vi "AUTOMAT.vi"() -> ()   [LabVIEW 2014]
uses:
  Timer 2013/Control Timer.ctl
  <vilib>/Platform/TimedLoop/XDataNode/timing_clust.ctl
  <vilib>/Platform/TimedLoop/XDataNode/nitl_modes.ctl
  <vilib>/Platform/TimedLoop/XDataNode/wakeup.ctl
  <vilib>/platform/TimedLoop/XDataNode/XDataNode.xnode
  <vilib>/Platform/TimedLoop/XDataNode/XDNodeRunTimeDep.lvlib
panel:
  out "Siren":bool
  out "B4":bool
  out "B1":bool
  out "B2":bool
  out "B3":bool
  out "B5":bool
  out "Ventil":bool
  out "SISTEM":bool
  out "PUMPE":bool
  out "Pump 2":bool
  out "Pump 1":bool
  in  "GENERAL STOP":bool
  in  "RUCNO/AUTOMATSKI":bool
  in  "Accept Stop":bool
  out "SYSTEM STOPPED":bool
  in  "Pumpe OFF":bool
  in  "Pumpe ON":bool
  in  "Sistem OFF":bool
  in  "Sistem ON":bool
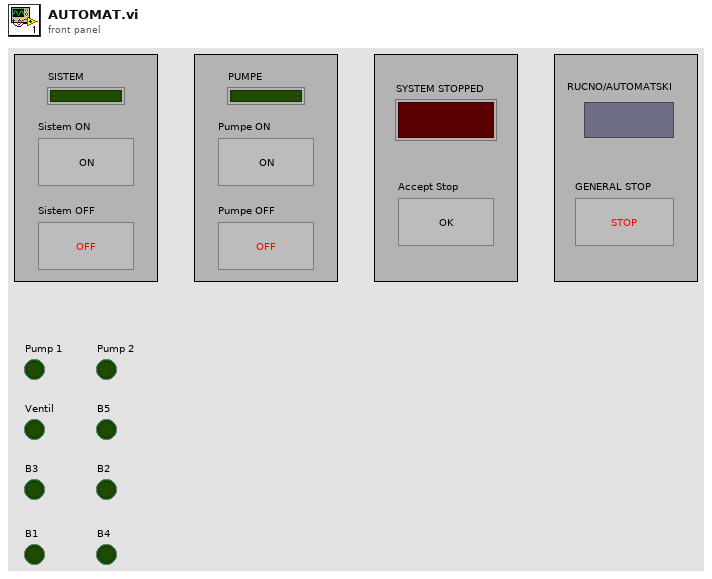
[diagram p1: front panel]
types:
  T1 = typedef "Control Timer.ctl" = enum16{"Timecheck", "Reset"}
  T2 = typedef "XDNodeRunTimeDep.lvlib/timing_clust.ctl" = cluster{"Expected End [f-1]":u64, "Actual End [f-1]":u64, "Finished Late? [f-1]":bool, "Expected End [i-1]":u64, "Actual End [i-1]":u64, "Finished Late? [i-1]":bool, "Expected Start [i]":u64, "Actual Start [i]":u64, "Expected Start [f]":u64, "Actual Start [f]":u64, "Source Name":string, "Structure Name":string, "Period":i64, "Deadline":i64, "Offset":i64, "Start":i64, "Priority":i32, "Timeout":i32, "Mode":T3, "Wakeup Reason":T4, "Error":errorcluster, "Source Type":string, "Secondary Source Type":string, "Global End Time":u64, "Global Start Time":u64, "Frame Duration":u64, "Iteration Duration":u64, "Assigned CPU":i32, "I/O Scan Engine Mode":u32}
  T3 = typedef "XDNodeRunTimeDep.lvlib/nitl_modes.ctl" = enum32{"No Change", "Process missed periods, maintain original phase", "Discard missed periods, maintain original phase", "Process missed periods, ignore original phase", "Discard missed periods, ignore original phase"}
  T4 = typedef "XDNodeRunTimeDep.lvlib/wakeup.ctl" = enum32{"Normal", "Aborted", "Asynchronous wakeup", "Timing source error", "Timed loop error", "Timeout"}
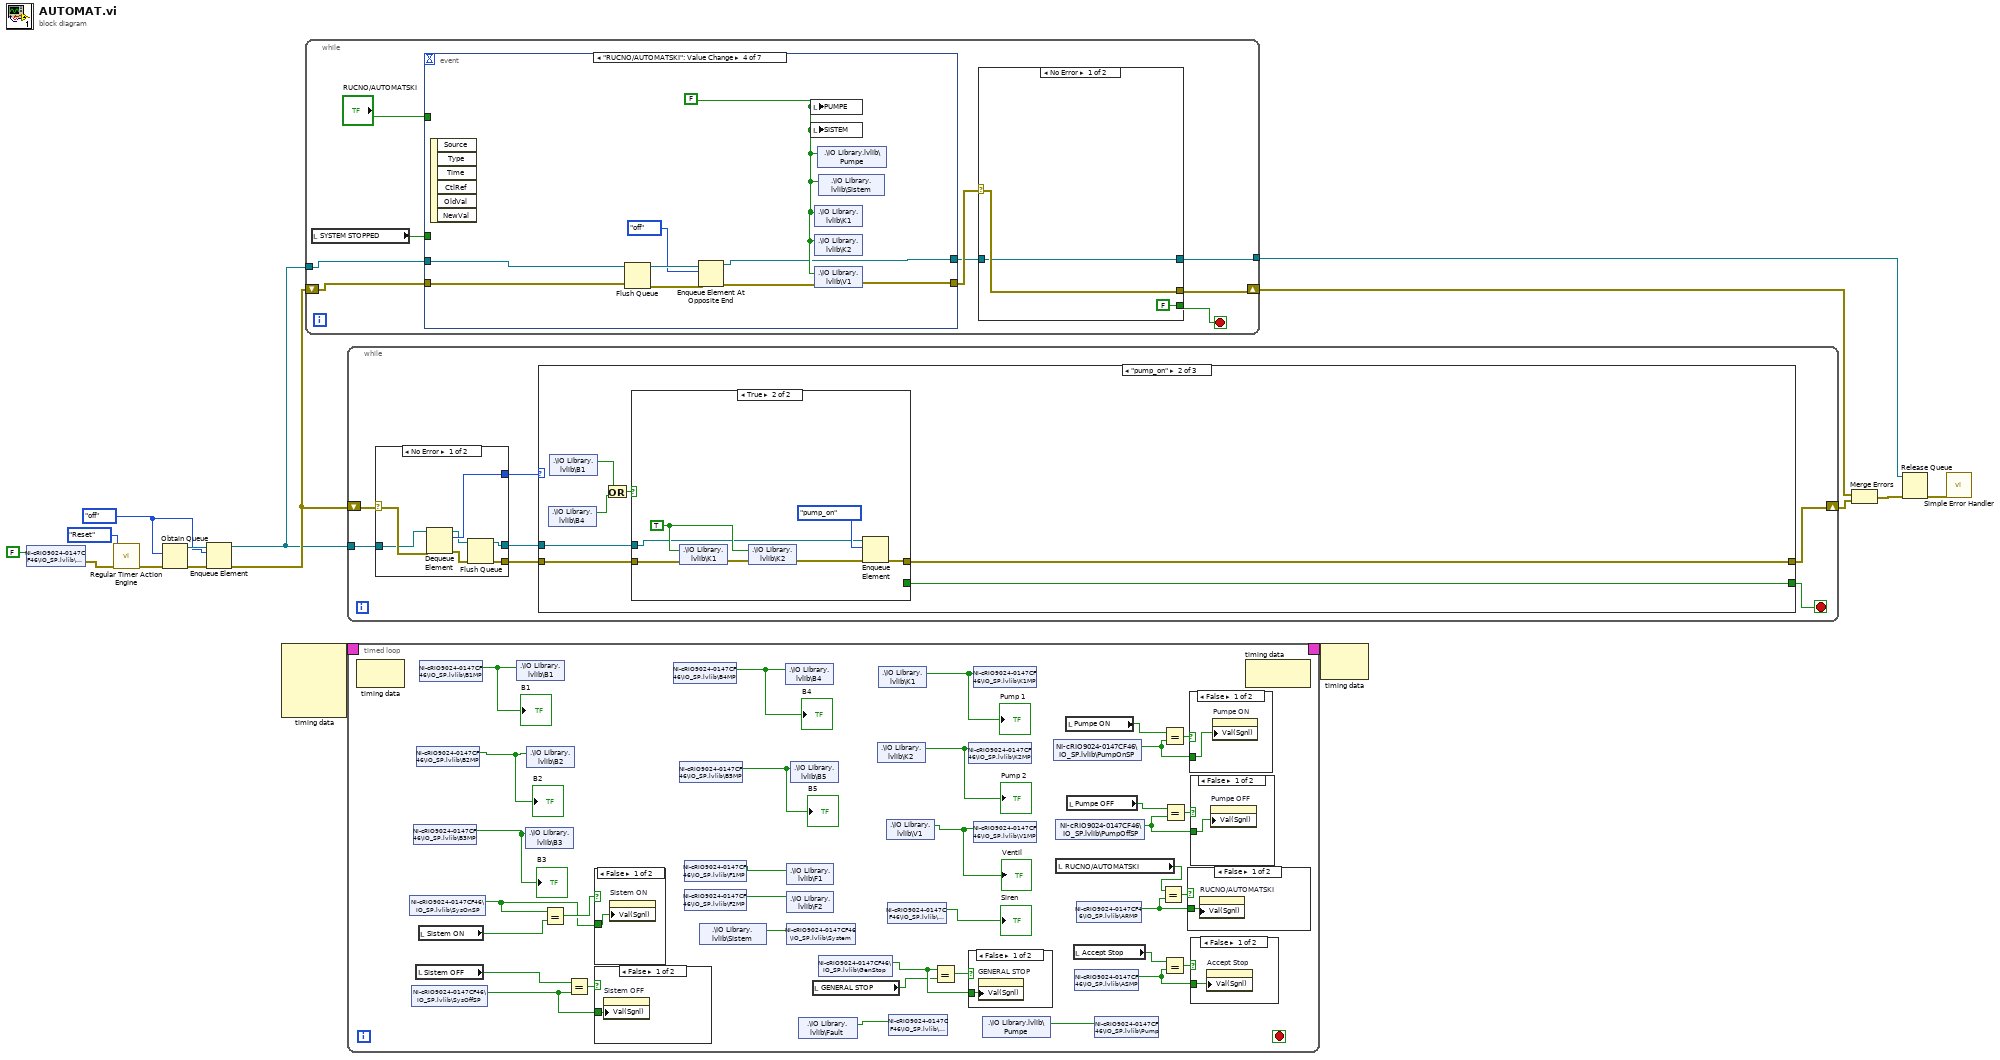
[diagram p0: block diagram]
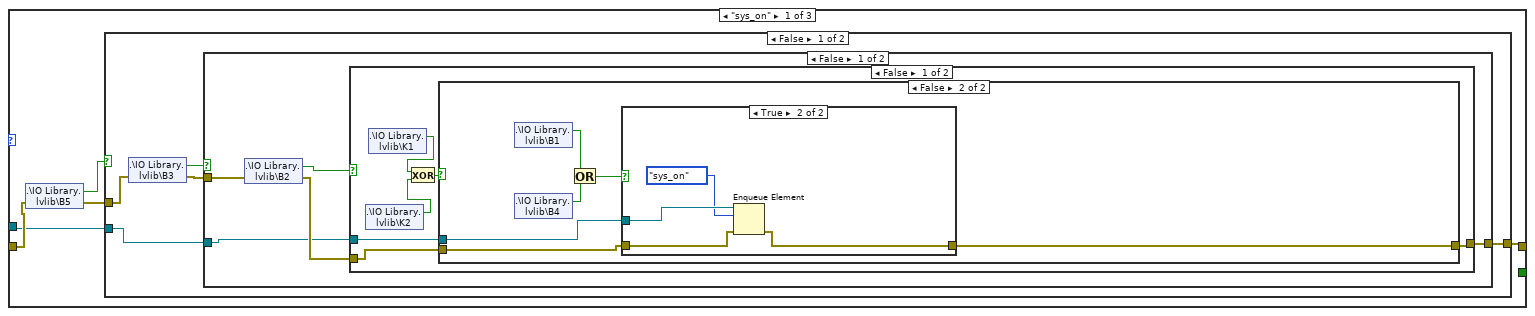
[diagram p9: hidden frame]
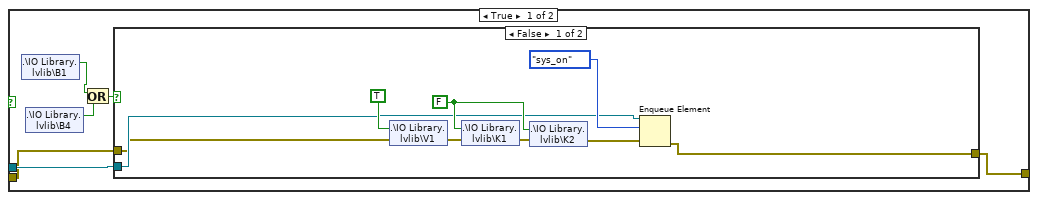
[diagram p10: hidden frame]
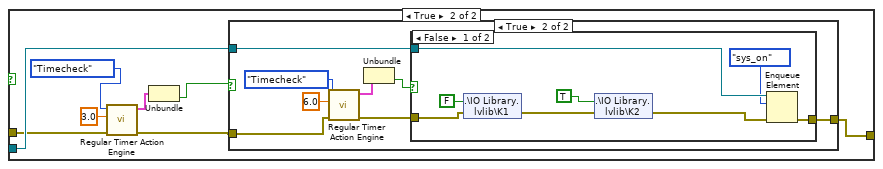
[diagram p11: hidden frame]
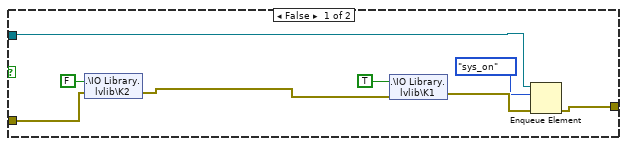
[diagram p12: hidden frame]
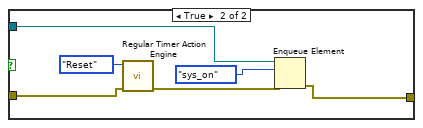
[diagram p13: hidden frame]
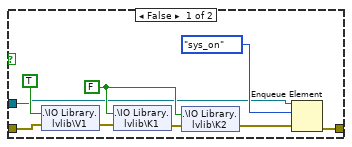
[diagram p14: hidden frame]
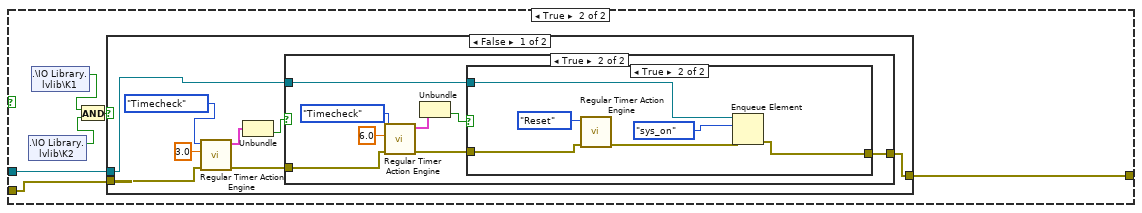
[diagram p15: hidden frame]
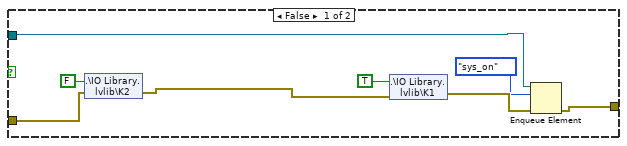
[diagram p16: hidden frame]
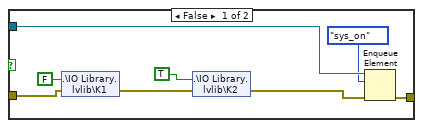
[diagram p17: hidden frame]
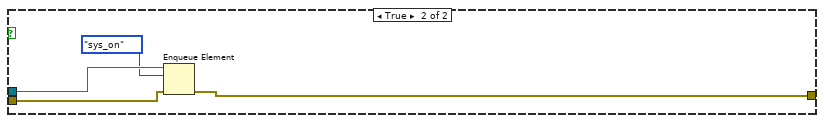
[diagram p18: hidden frame]
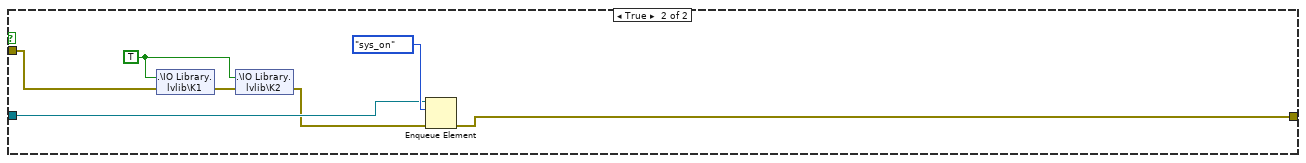
[diagram p19: hidden frame]
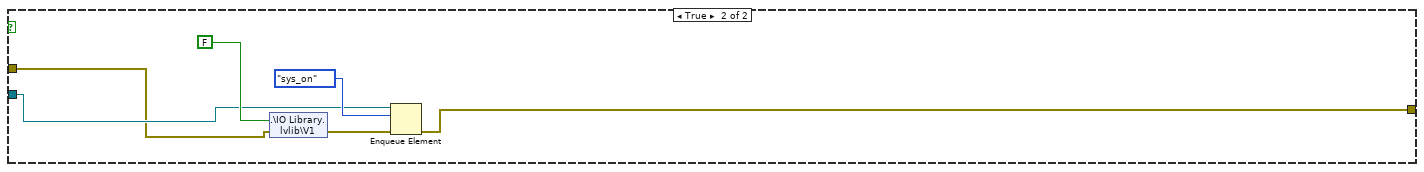
[diagram p20: hidden frame]
diagram:
  w14 = enum16{"sys_on", "pump_on", "off"}."off" ("Enum")
  n1 = shared-variable "NI-cRIO9024-0147CF46\\IO_SP.lvlib\\Siren"(FALSE ("Siren")) -> (error out=w2:errorcluster)  [unwired: 1 in]
  n2 = call "Regular Timer Action Engine.vi"("Enum"=Control_Timer."Reset", "error in"=w2) -> ("error out"=w11:errorcluster)  [unwired: 7 in, 1 out]
  n3 = Obtain Queue(element data type=w14, error in (no error)=w11) -> (queue out=w15:refnum<queue>, error out=w16:errorcluster)  [unwired: 3 in, 1 out]
  n4 = Enqueue Element(queue=w15, element=w14, error in (no error)=w16) -> (queue out=w12:refnum<queue>, error out=w13:errorcluster)  [unwired: 1 in, 1 out]
  n5 = node-c288() -> (w4:T2)  [unwired: 4 in]
  n6 = while {
    tunnel: w12 -> [w17]
    shift-right: [w25] -> w8
    shift-left: w13 -> [w18]
    tunnel: [w20] -> w9
    stop <- w24 stop-if-true
    n7 = local read "SYSTEM STOPPED"() -> (w21:bool)
    n8 = event shown="[3] \"RUCNO/AUTOMATSKI\": Value Change" {
      selector: _ -> [_ _ _ _ _ _ _]
      dyn-events: _ -> [_ _ _ _ _ _ _]
      timeout: _ -> [_ _ _ _ _ _ _]
      tunnel: "RUCNO/AUTOMATSKI" -> [w31 _ _ _ w85 w109 w126]
      tunnel: w18 -> [w30 w51 w61 w79 w83 w107 w124]
      tunnel: w17 -> [w29 w49 w70 w78 w82 w106 w125]
      tunnel: [w28 w52 w64 w77 w84 w108 w123] -> w22
      tunnel: w21 -> [w27 _ _ _ w81 _ _]
      tunnel: [w26 w50 w66 w73 w80 w105 w122] -> w19
      event "Pumpe ON": Value Change {
        n9 = event-data() -> ()  [unwired: 1 in, 6 out]
        n10 = case shown="False" w27 {
          tunnel: w31 -> [_ w38]
          tunnel: w30 -> [w33 w37]
          tunnel: w29 -> [w32 w36]
          tunnel: [w33 w35] -> w28
          tunnel: [w32 w34] -> w26
          frame True {
          }
          frame False {
            n11 = case shown="False" w38 {
              tunnel: w37 -> [w39 w48]
              tunnel: w36 -> [w40 w47]
              tunnel: [w39 w44] -> w35
              tunnel: [w40 w45] -> w34
              frame True {
              }
              frame False {
                w46 = TRUE ("Pump 2 contactor")
                n12 = Flush Queue(queue=w47, error in (no error)=w48) -> (queue out=w42:refnum<queue>, error out=w41:errorcluster)  [unwired: 1 out]
                n13 = shared-variable ".\\IO Library.lvlib\\K1"(w46) -> ()  [unwired: 1 in, 1 out]
                n14 = shared-variable ".\\IO Library.lvlib\\K2"(w46) -> ()  [unwired: 1 in, 1 out]
                n15 = shared-variable ".\\IO Library.lvlib\\Pumpe"(w46) -> ()  [unwired: 1 in, 1 out]
                n16 = Enqueue Element At Opposite End(queue=w42, element=enum16{"sys_on", "pump_on", "off"}."pump_on", error in (no error)=w41) -> (queue out=w45:refnum<queue>, error out=w44:errorcluster)  [unwired: 1 in, 1 out]
                "PUMPE" <- w46
              }
            }
          }
        }
      }
      event "Accept Stop": Value Change {
        n17 = event-data() -> ()  [unwired: 1 in, 6 out]
        n18 = local read "GENERAL STOP"() -> (w53:bool)
        n19 = case shown="False" w53 {
          tunnel: [w54 w59] -> w52
          tunnel: w51 -> [w55 w59]
          tunnel: [w57 w58] -> w50
          tunnel: w49 -> [w57 w58]
          frame False {
            w56 = FALSE ("SYSTEM STOPPED")
            n20 = shared-variable ".\\IO Library.lvlib\\Fault"(w56, error in=w55) -> (error out=w54:errorcluster)
            "SYSTEM STOPPED" <- w56
          }
          frame True {
          }
        }
      }
      event "GENERAL STOP": Value Change {
        w60 = FALSE
        w63 = TRUE ("SYSTEM STOPPED")
        n21 = event-data() -> ()  [unwired: 1 in, 6 out]
        n22 = shared-variable ".\\IO Library.lvlib\\Fault"(w63, error in=w61) -> (error out=w62:errorcluster)
        n23 = local write "SYSTEM STOPPED"(w63) -> ()
        n24 = Flush Queue(queue=w70, error in (no error)=w62) -> (queue out=w68:refnum<queue>, error out=w69:errorcluster)  [unwired: 1 out]
        n25 = Enqueue Element At Opposite End(queue=w68, element=enum16{"sys_on", "pump_on", "off"}."off", error in (no error)=w69) -> (queue out=w66:refnum<queue>, error out=w65:errorcluster)  [unwired: 1 in, 1 out]
        n26 = shared-variable ".\\IO Library.lvlib\\Pumpe"(w60) -> ()  [unwired: 1 in, 1 out]
        n27 = shared-variable ".\\IO Library.lvlib\\Sistem"(w60) -> ()  [unwired: 1 in, 1 out]
        n28 = local write "SISTEM"(w60) -> ()
        n29 = local write "PUMPE"(w60) -> ()
        n30 = shared-variable ".\\IO Library.lvlib\\K1"(w60) -> ()  [unwired: 1 in, 1 out]
        n31 = shared-variable ".\\IO Library.lvlib\\K2"(w60) -> ()  [unwired: 1 in, 1 out]
        n32 = shared-variable ".\\IO Library.lvlib\\V1"(w60) -> ()  [unwired: 1 in, 1 out]
        n33 = shared-variable "NI-cRIO9024-0147CF46\\IO_SP.lvlib\\Siren"(w60, error in=w65) -> (error out=w64:errorcluster)
      }
      event "RUCNO/AUTOMATSKI": Value Change {
        w76 = FALSE
        n34 = event-data() -> ()  [unwired: 1 in, 6 out]
        n35 = Flush Queue(queue=w78, error in (no error)=w79) -> (queue out=w74:refnum<queue>, error out=w75:errorcluster)  [unwired: 1 out]
        n36 = Enqueue Element At Opposite End(queue=w74, element=enum16{"sys_on", "pump_on", "off"}."off", error in (no error)=w75) -> (queue out=w73:refnum<queue>, error out=w72:errorcluster)  [unwired: 1 in, 1 out]
        n37 = local write "PUMPE"(w76) -> ()
        n38 = local write "SISTEM"(w76) -> ()
        n39 = shared-variable ".\\IO Library.lvlib\\K1"(w76) -> ()  [unwired: 1 in, 1 out]
        n40 = shared-variable ".\\IO Library.lvlib\\K2"(w76) -> ()  [unwired: 1 in, 1 out]
        n41 = shared-variable ".\\IO Library.lvlib\\V1"(w76, error in=w72) -> (error out=w77:errorcluster)
        n42 = shared-variable ".\\IO Library.lvlib\\Pumpe"(w76) -> ()  [unwired: 1 in, 1 out]
        n43 = shared-variable ".\\IO Library.lvlib\\Sistem"(w76) -> ()  [unwired: 1 in, 1 out]
      }
      event "Sistem ON": Value Change {
        n44 = event-data() -> ()  [unwired: 1 in, 6 out]
        n45 = case shown="False" w81 {
          tunnel: w85 -> [_ w92]
          tunnel: [w87 w91] -> w84
          tunnel: w83 -> [w87 w90]
          tunnel: w82 -> [w86 w89]
          tunnel: [w86 w88] -> w80
          frame True {
          }
          frame False {
            n46 = case shown="True" w92 {
              tunnel: [w93 w99] -> w91
              tunnel: w90 -> [w93 w95]
              tunnel: w89 -> [w94 w98]
              tunnel: [w94 w100] -> w88
              frame False {
              }
              frame True {
                w97 = TRUE ("V1")
                n47 = shared-variable ".\\IO Library.lvlib\\Sistem"(w97, error in=w95) -> (error out=w96:errorcluster)
                n48 = shared-variable ".\\IO Library.lvlib\\V1"(w97, error in=w96) -> (error out=w104:errorcluster)
                n49 = Flush Queue(queue=w98, error in (no error)=w104) -> (queue out=w102:refnum<queue>, error out=w103:errorcluster)  [unwired: 1 out]
                n50 = Enqueue Element At Opposite End(queue=w102, element=enum16{"sys_on", "pump_on", "off"}."sys_on", error in (no error)=w103) -> (queue out=w100:refnum<queue>, error out=w99:errorcluster)  [unwired: 1 in, 1 out]
                "SISTEM" <- w97
              }
            }
          }
        }
      }
      event "Sistem OFF": Value Change {
        n51 = event-data() -> ()  [unwired: 1 in, 6 out]
        n52 = case shown="True" w109 {
          tunnel: [w110 w116] -> w108
          tunnel: w107 -> [w110 w112]
          tunnel: w106 -> [w111 w115]
          tunnel: [w111 w117] -> w105
          frame False {
          }
          frame True {
            w114 = FALSE ("V1")
            n53 = shared-variable ".\\IO Library.lvlib\\Sistem"(w114, error in=w112) -> (error out=w113:errorcluster)
            n54 = local write "SISTEM"(w114) -> ()
            n55 = shared-variable ".\\IO Library.lvlib\\V1"(w114, error in=w113) -> (error out=w121:errorcluster)
            n56 = Flush Queue(queue=w115, error in (no error)=w121) -> (queue out=w119:refnum<queue>, error out=w120:errorcluster)  [unwired: 1 out]
            n57 = Enqueue Element At Opposite End(queue=w119, element=enum16{"sys_on", "pump_on", "off"}."off", error in (no error)=w120) -> (queue out=w117:refnum<queue>, error out=w116:errorcluster)  [unwired: 1 in, 1 out]
          }
        }
      }
      event "Pumpe OFF": Value Change {
        n58 = event-data() -> ()  [unwired: 1 in, 6 out]
        n59 = case shown="False" w126 {
          tunnel: w125 -> [w128 w134]
          tunnel: w124 -> [w127 w135]
          tunnel: [w127 w133] -> w123
          tunnel: [w128 w132] -> w122
          frame True {
          }
          frame False {
            w129 = FALSE ("Pump 1 contactor")
            n60 = Flush Queue(queue=w134, error in (no error)=w135) -> (queue out=w137:refnum<queue>, error out=w138:errorcluster)  [unwired: 1 out]
            n61 = Enqueue Element At Opposite End(queue=w137, element=enum16{"sys_on", "pump_on", "off"}."off", error in (no error)=w138) -> (queue out=w132:refnum<queue>, error out=w136:errorcluster)  [unwired: 1 in, 1 out]
            n62 = local write "PUMPE"(FALSE ("PUMPE")) -> ()
            n63 = shared-variable ".\\IO Library.lvlib\\K1"(w129, error in=w136) -> (error out=w131:errorcluster)
            n64 = shared-variable ".\\IO Library.lvlib\\Pumpe"(w129, error in=w131) -> (error out=w130:errorcluster)
            n65 = shared-variable ".\\IO Library.lvlib\\K2"(w129, error in=w130) -> (error out=w133:errorcluster)
          }
        }
      }
    }
    n66 = case shown="No Error" w22 {
      selector: w22 -> [w143 w146]
      tunnel: [w143 w146] -> w25
      tunnel: [FALSE TRUE] -> w24
      tunnel: [w141 w144] -> w20
      tunnel: w19 -> [w141 w144]
      frame No Error {
      }
      frame Error {
      }
    }
  }
  n67 = while {
    shift-right: [w148] -> w7
    shift-left: w13 -> [w153]
    tunnel: w12 -> [w152]
    stop <- w147 stop-if-true
    n68 = case shown="No Error" w153 {
      selector: w153 -> [w342 w345]
      tunnel: w152 -> [w341 w343]
      tunnel: [w340 enum16{"sys_on", "pump_on", "off"}."off" ("Enum")] -> w151
      tunnel: [w339 w345] -> w150
      tunnel: [w338 w343] -> w149
      frame No Error {
        n69 = Dequeue Element(queue=w341, error in (no error)=w342) -> (queue out=w337:refnum<queue>, element=w340:enum16{"sys_on", "pump_on", "off"}, error out=w336:errorcluster)  [unwired: 1 in, 1 out]
        n70 = Flush Queue(queue=w337, error in (no error)=w336) -> (queue out=w338:refnum<queue>, error out=w339:errorcluster)  [unwired: 1 out]
      }
      frame Error {
      }
    }
    n71 = case shown="\"pump_on\"" w151 {
      tunnel: [w155 w313 w332] -> w148
      tunnel: w150 -> [w157 w312 w328]
      tunnel: w149 -> [w154 w309 w331]
      tunnel: [_ w308 _] -> w147
      frame "sys_on" {
        n72 = shared-variable ".\\IO Library.lvlib\\B5"(error in=w157) -> (w158:bool, error out=w156:errorcluster)
        n73 = case shown="False" w158 {
          tunnel: w156 -> [w163 w303]
          tunnel: [w161 w302] -> w155
          tunnel: w154 -> [w160 w304]
          frame False {
            n74 = shared-variable ".\\IO Library.lvlib\\B3"(error in=w163) -> (w162:bool, error out=w159:errorcluster)
            n75 = case shown="False" w162 {
              tunnel: [w166 w300] -> w161
              tunnel: w160 -> [w164 w299]
              tunnel: w159 -> [w167 w298]
              frame False {
                n76 = shared-variable ".\\IO Library.lvlib\\B2"(error in=w167) -> (w168:bool, error out=w165:errorcluster)
                n77 = case shown="False" w168 {
                  tunnel: [w174 w248] -> w166
                  tunnel: w165 -> [w172 w249]
                  tunnel: w164 -> [w173 w247]
                  frame False {
                    n78 = shared-variable ".\\IO Library.lvlib\\K2"() -> (w169:bool)  [unwired: 1 in, 1 out]
                    n79 = shared-variable ".\\IO Library.lvlib\\K1"() -> (w170:bool)  [unwired: 1 in, 1 out]
                    n80 = Exclusive Or(1:w169, 2:w170) -> (0:w171:bool)
                    n81 = case shown="False" w171 {
                      tunnel: [w180 w230] -> w174
                      tunnel: w173 -> [w176 w229]
                      tunnel: w172 -> [w175 w228]
                      frame True {
                        n82 = shared-variable ".\\IO Library.lvlib\\B1"() -> (w178:bool)  [unwired: 1 in, 1 out]
                        n83 = shared-variable ".\\IO Library.lvlib\\B4"() -> (w177:bool)  [unwired: 1 in, 1 out]
                        n84 = Or(x=w178, y=w177) -> (x .or. y?=w179:bool)
                        n85 = case shown="False" w179 {
                          tunnel: [w181 w192] -> w180
                          tunnel: w176 -> [w186 w191]
                          tunnel: w175 -> [w185 w190]
                          frame False {
                            w187 = FALSE
                            n86 = shared-variable ".\\IO Library.lvlib\\V1"(TRUE, error in=w185) -> (error out=w184:errorcluster)
                            n87 = shared-variable ".\\IO Library.lvlib\\K1"(w187, error in=w184) -> (error out=w183:errorcluster)
                            n88 = shared-variable ".\\IO Library.lvlib\\K2"(w187, error in=w183) -> (error out=w182:errorcluster)
                            n89 = Enqueue Element(queue=w186, element=enum16{"sys_on", "pump_on", "off"}."sys_on", error in (no error)=w182) -> (error out=w181:errorcluster)  [unwired: 1 in, 2 out]
                          }
                          frame True {
                            n90 = call "Regular Timer Action Engine.vi"("Enum"=Control_Timer."Timecheck", "Time Target"=3.0, "error in"=w190) -> ("Status"=w195:cluster{"Running":bool, "Done":bool}, "error out"=w193:errorcluster)  [unwired: 6 in]
                            n91 = Unbundle(w195) -> ("Done"=w194:bool)  [unwired: 1 out]
                            n92 = case shown="True" w194 {
                              tunnel: w193 -> [w204 w211]
                              tunnel: [w203 w207] -> w192
                              tunnel: w191 -> [w201 w206]
                              frame False {
                                n93 = shared-variable ".\\IO Library.lvlib\\K2"(FALSE ("F2"), error in=w204) -> (error out=w199:errorcluster)
                                n94 = shared-variable ".\\IO Library.lvlib\\K1"(TRUE ("Pump 2 contactor"), error in=w199) -> (error out=w202:errorcluster)
                                n95 = Enqueue Element(queue=w201, element=enum16{"sys_on", "pump_on", "off"}."sys_on", error in (no error)=w202) -> (error out=w203:errorcluster)  [unwired: 1 in, 2 out]
                              }
                              frame True {
                                n96 = call "Regular Timer Action Engine.vi"("Enum"=Control_Timer."Timecheck", "Time Target"=6.0, "error in"=w211) -> ("Status"=w210:cluster{"Running":bool, "Done":bool}, "error out"=w208:errorcluster)  [unwired: 6 in]
                                n97 = Unbundle(w210) -> ("Done"=w209:bool)  [unwired: 1 out]
                                n98 = case shown="False" w209 {
                                tunnel: w208 -> [w216 w227]
                                tunnel: [w220 w224] -> w207
                                tunnel: w206 -> [w219 w223]
                                frame False {
                                n99 = shared-variable ".\\IO Library.lvlib\\K1"(FALSE ("K1"), error in=w216) -> (error out=w215:errorcluster)
                                n100 = shared-variable ".\\IO Library.lvlib\\K2"(TRUE ("Pump 2 contactor"), error in=w215) -> (error out=w214:errorcluster)
                                n101 = Enqueue Element(queue=w219, element=enum16{"sys_on", "pump_on", "off"}."sys_on", error in (no error)=w214) -> (error out=w220:errorcluster)  [unwired: 1 in, 2 out]
                                }
                                frame True {
                                n102 = call "Regular Timer Action Engine.vi"("Enum"=Control_Timer."Reset", "error in"=w227) -> ("error out"=w225:errorcluster)  [unwired: 7 in, 1 out]
                                n103 = Enqueue Element(queue=w223, element=enum16{"sys_on", "pump_on", "off"}."sys_on", error in (no error)=w225) -> (error out=w224:errorcluster)  [unwired: 1 in, 2 out]
                                }
                                }
                              }
                            }
                          }
                        }
                      }
                      frame False {
                        n104 = shared-variable ".\\IO Library.lvlib\\B1"() -> (w232:bool)  [unwired: 1 in, 1 out]
                        n105 = shared-variable ".\\IO Library.lvlib\\B4"() -> (w231:bool)  [unwired: 1 in, 1 out]
                        n106 = Or(x=w232, y=w231) -> (x .or. y?=w233:bool)
                        n107 = case shown="True" w233 {
                          tunnel: w228 -> [w240 w246]
                          tunnel: [w242 w245] -> w230
                          tunnel: w229 -> [w234 w244]
                          frame False {
                            w235 = FALSE
                            n108 = shared-variable ".\\IO Library.lvlib\\V1"(TRUE, error in=w240) -> (error out=w238:errorcluster)
                            n109 = shared-variable ".\\IO Library.lvlib\\K1"(w235, error in=w238) -> (error out=w236:errorcluster)
                            n110 = shared-variable ".\\IO Library.lvlib\\K2"(w235, error in=w236) -> (error out=w237:errorcluster)
                            n111 = Enqueue Element(queue=w234, element=enum16{"sys_on", "pump_on", "off"}."sys_on", error in (no error)=w237) -> (error out=w242:errorcluster)  [unwired: 1 in, 2 out]
                          }
                          frame True {
                            n112 = Enqueue Element(queue=w244, element=enum16{"sys_on", "pump_on", "off"}."sys_on", error in (no error)=w246) -> (error out=w245:errorcluster)  [unwired: 1 in, 2 out]
                          }
                        }
                      }
                    }
                  }
                  frame True {
                    n113 = shared-variable ".\\IO Library.lvlib\\K2"() -> (w250:bool)  [unwired: 1 in, 1 out]
                    n114 = shared-variable ".\\IO Library.lvlib\\K1"() -> (w251:bool)  [unwired: 1 in, 1 out]
                    n115 = And(x=w251, y=w250) -> (x .and. y?=w252:bool)
                    n116 = case shown="False" w252 {
                      tunnel: w249 -> [w257 w294]
                      tunnel: [w254 w293] -> w248
                      tunnel: w247 -> [w253 w292]
                      frame False {
                        n117 = call "Regular Timer Action Engine.vi"("Enum"=Control_Timer."Timecheck", "Time Target"=3.0, "error in"=w257) -> ("Status"=w258:cluster{"Running":bool, "Done":bool}, "error out"=w255:errorcluster)  [unwired: 6 in]
                        n118 = Unbundle(w258) -> ("Done"=w256:bool)  [unwired: 1 out]
                        n119 = case shown="True" w256 {
                          tunnel: w255 -> [w267 w274]
                          tunnel: [w266 w270] -> w254
                          tunnel: w253 -> [w264 w269]
                          frame False {
                            n120 = shared-variable ".\\IO Library.lvlib\\K2"(FALSE ("F2"), error in=w267) -> (error out=w262:errorcluster)
                            n121 = shared-variable ".\\IO Library.lvlib\\K1"(TRUE ("Pump 2 contactor"), error in=w262) -> (error out=w265:errorcluster)
                            n122 = Enqueue Element(queue=w264, element=enum16{"sys_on", "pump_on", "off"}."sys_on", error in (no error)=w265) -> (error out=w266:errorcluster)  [unwired: 1 in, 2 out]
                          }
                          frame True {
                            n123 = call "Regular Timer Action Engine.vi"("Enum"=Control_Timer."Timecheck", "Time Target"=6.0, "error in"=w274) -> ("Status"=w273:cluster{"Running":bool, "Done":bool}, "error out"=w271:errorcluster)  [unwired: 6 in]
                            n124 = Unbundle(w273) -> ("Done"=w272:bool)  [unwired: 1 out]
                            n125 = case shown="True" w272 {
                              tunnel: w271 -> [w279 w290]
                              tunnel: [w283 w287] -> w270
                              tunnel: w269 -> [w282 w286]
                              frame False {
                                n126 = shared-variable ".\\IO Library.lvlib\\K1"(FALSE ("K1"), error in=w279) -> (error out=w278:errorcluster)
                                n127 = shared-variable ".\\IO Library.lvlib\\K2"(TRUE ("Pump 2 contactor"), error in=w278) -> (error out=w277:errorcluster)
                                n128 = Enqueue Element(queue=w282, element=enum16{"sys_on", "pump_on", "off"}."sys_on", error in (no error)=w277) -> (error out=w283:errorcluster)  [unwired: 1 in, 2 out]
                              }
                              frame True {
                                n129 = call "Regular Timer Action Engine.vi"("Enum"=Control_Timer."Reset", "error in"=w290) -> ("error out"=w288:errorcluster)  [unwired: 7 in, 1 out]
                                n130 = Enqueue Element(queue=w286, element=enum16{"sys_on", "pump_on", "off"}."sys_on", error in (no error)=w288) -> (error out=w287:errorcluster)  [unwired: 1 in, 2 out]
                              }
                            }
                          }
                        }
                      }
                      frame True {
                        n131 = Enqueue Element(queue=w292, element=enum16{"sys_on", "pump_on", "off"}."sys_on", error in (no error)=w294) -> (error out=w293:errorcluster)  [unwired: 1 in, 2 out]
                      }
                    }
                  }
                }
              }
              frame True {
                w295 = TRUE ("x")
                n132 = shared-variable ".\\IO Library.lvlib\\K1"(w295, error in=w298) -> (error out=w297:errorcluster)
                n133 = shared-variable ".\\IO Library.lvlib\\K2"(w295, error in=w297) -> (error out=w296:errorcluster)
                n134 = Enqueue Element(queue=w299, element=enum16{"sys_on", "pump_on", "off"}."sys_on", error in (no error)=w296) -> (error out=w300:errorcluster)  [unwired: 1 in, 2 out]
              }
            }
          }
          frame True {
            n135 = shared-variable ".\\IO Library.lvlib\\V1"(FALSE ("V1"), error in=w303) -> (error out=w307:errorcluster)
            n136 = Enqueue Element(queue=w304, element=enum16{"sys_on", "pump_on", "off"}."sys_on", error in (no error)=w307) -> (error out=w302:errorcluster)  [unwired: 1 in, 2 out]
          }
        }
      }
      frame "pump_on" {
        n137 = shared-variable ".\\IO Library.lvlib\\B4"() -> (w310:bool)  [unwired: 1 in, 1 out]
        n138 = shared-variable ".\\IO Library.lvlib\\B1"() -> (w311:bool)  [unwired: 1 in, 1 out]
        n139 = Or(x=w311, y=w310) -> (x .or. y?=w314:bool)
        n140 = case shown="True" w314 {
          tunnel: [w317 w325] -> w313
          tunnel: w312 -> [w316 w322]
          tunnel: w309 -> [_ w319]
          tunnel: [FALSE _] -> w308
          frame False {
            n141 = shared-variable "NI-cRIO9024-0147CF46\\IO_SP.lvlib\\Siren"(TRUE ("Siren"), error in=w316) -> (error out=w317:errorcluster)
          }
          frame True {
            w323 = TRUE
            n142 = shared-variable ".\\IO Library.lvlib\\K1"(w323, error in=w322) -> (error out=w321:errorcluster)
            n143 = shared-variable ".\\IO Library.lvlib\\K2"(w323, error in=w321) -> (error out=w320:errorcluster)
            n144 = Enqueue Element(queue=w319, element=enum16{"sys_on", "pump_on", "off"}."pump_on", error in (no error)=w320) -> (error out=w325:errorcluster)  [unwired: 1 in, 2 out]
          }
        }
      }
      frame "off", Default {
        n145 = shared-variable ".\\IO Library.lvlib\\K1"(FALSE ("K1"), error in=w328) -> (error out=w327:errorcluster)
        n146 = shared-variable ".\\IO Library.lvlib\\K2"(FALSE ("K2"), error in=w327) -> (error out=w326:errorcluster)
        n147 = shared-variable ".\\IO Library.lvlib\\V1"(FALSE ("V1"), error in=w326) -> (error out=w329:errorcluster)
        n148 = Enqueue Element(queue=w331, element=enum16{"sys_on", "pump_on", "off"}."off", error in (no error)=w329) -> (error out=w332:errorcluster)  [unwired: 1 in, 2 out]
      }
    }
  }
  n149 = timed-loop {
    timing: w4 -> [_]
    timing-out: [_] -> w3
    stop <- _ stop-if-true
    n150 = node-c288() -> ()  [unwired: 1 in, 1 out]
    n151 = shared-variable "NI-cRIO9024-0147CF46\\IO_SP.lvlib\\SysOnSP"() -> (w377:bool)  [unwired: 1 in, 1 out]
    n152 = shared-variable "NI-cRIO9024-0147CF46\\IO_SP.lvlib\\SysOffSP"() -> (w371:bool)  [unwired: 1 in, 1 out]
    n153 = shared-variable "NI-cRIO9024-0147CF46\\IO_SP.lvlib\\B3MP"() -> (w349:bool)  [unwired: 1 in, 1 out]
    "B3" <- w349
    n154 = local read "Sistem OFF"() -> (w370:bool)
    n155 = shared-variable "NI-cRIO9024-0147CF46\\IO_SP.lvlib\\B2MP"() -> (w350:bool)  [unwired: 1 in, 1 out]
    "B2" <- w350
    n156 = local read "Sistem ON"() -> (w379:bool)
    n157 = shared-variable "NI-cRIO9024-0147CF46\\IO_SP.lvlib\\B1MP"() -> (w351:bool)  [unwired: 1 in, 1 out]
    "B1" <- w351
    n158 = shared-variable ".\\IO Library.lvlib\\B1"(w351) -> ()  [unwired: 1 in, 1 out]
    n159 = shared-variable ".\\IO Library.lvlib\\B3"(w349) -> ()  [unwired: 1 in, 1 out]
    n160 = shared-variable ".\\IO Library.lvlib\\B2"(w350) -> ()  [unwired: 1 in, 1 out]
    n161 = Equal?(x=w377, y=w379) -> (x = y?=w378:bool)
    n162 = Equal?(x=w370, y=w371) -> (x = y?=w372:bool)
    n163 = case shown="False" w378 {
      tunnel: w377 -> [w387 _]
      frame False {
        n164 = property on="Sistem ON" class="Bool (strict)"("Val(Sgnl)"=w387) -> ()  [unwired: 2 in, 2 out]
      }
      frame True {
      }
    }
    n165 = case shown="False" w372 {
      tunnel: w371 -> [w385 _]
      frame False {
        n166 = property on="Sistem OFF" class="Bool (strict)"("Val(Sgnl)"=w385) -> ()  [unwired: 2 in, 2 out]
      }
      frame True {
      }
    }
    n167 = shared-variable "NI-cRIO9024-0147CF46\\IO_SP.lvlib\\B4MP"() -> (w352:bool)  [unwired: 1 in, 1 out]
    "B4" <- w352
    n168 = shared-variable "NI-cRIO9024-0147CF46\\IO_SP.lvlib\\B5MP"() -> (w353:bool)  [unwired: 1 in, 1 out]
    "B5" <- w353
    n169 = shared-variable "NI-cRIO9024-0147CF46\\IO_SP.lvlib\\F1MP"() -> (w357:bool)  [unwired: 1 in, 1 out]
    n170 = shared-variable "NI-cRIO9024-0147CF46\\IO_SP.lvlib\\F2MP"() -> (w356:bool)  [unwired: 1 in, 1 out]
    n171 = shared-variable ".\\IO Library.lvlib\\Sistem"() -> (w346:bool)  [unwired: 1 in, 1 out]
    n172 = shared-variable ".\\IO Library.lvlib\\B4"(w352) -> ()  [unwired: 1 in, 1 out]
    n173 = shared-variable ".\\IO Library.lvlib\\F1"(w357) -> ()  [unwired: 1 in, 1 out]
    n174 = shared-variable ".\\IO Library.lvlib\\F2"(w356) -> ()  [unwired: 1 in, 1 out]
    n175 = shared-variable "NI-cRIO9024-0147CF46\\IO_SP.lvlib\\System"(w346) -> ()  [unwired: 1 in, 1 out]
    n176 = shared-variable ".\\IO Library.lvlib\\B5"(w353) -> ()  [unwired: 1 in, 1 out]
    n177 = shared-variable ".\\IO Library.lvlib\\Fault"() -> (w348:bool)  [unwired: 1 in, 1 out]
    n178 = local read "GENERAL STOP"() -> (w373:bool)
    n179 = shared-variable "NI-cRIO9024-0147CF46\\IO_SP.lvlib\\GenStop"() -> (w374:bool)  [unwired: 1 in, 1 out]
    n180 = shared-variable ".\\IO Library.lvlib\\K2"() -> (w354:bool)  [unwired: 1 in, 1 out]
    "Pump 2" <- w354
    n181 = shared-variable ".\\IO Library.lvlib\\K1"() -> (w355:bool)  [unwired: 1 in, 1 out]
    "Pump 1" <- w355
    n182 = shared-variable ".\\IO Library.lvlib\\V1"() -> (w380:bool)  [unwired: 1 in, 1 out]
    "Ventil" <- w380
    n183 = shared-variable "NI-cRIO9024-0147CF46\\IO_SP.lvlib\\Siren"() -> (→"Siren":bool)  [unwired: 1 in, 1 out]
    n184 = shared-variable "NI-cRIO9024-0147CF46\\IO_SP.lvlib\\Fault"(w348) -> ()  [unwired: 1 in, 1 out]
    n185 = Equal?(x=w374, y=w373) -> (x = y?=w375:bool)
    n186 = case shown="False" w375 {
      tunnel: w374 -> [w386 _]
      frame False {
        n187 = property on="GENERAL STOP" class="Bool (strict)"("Val(Sgnl)"=w386) -> ()  [unwired: 2 in, 2 out]
      }
      frame True {
      }
    }
    n188 = shared-variable "NI-cRIO9024-0147CF46\\IO_SP.lvlib\\K2MP"(w354) -> ()  [unwired: 1 in, 1 out]
    n189 = shared-variable "NI-cRIO9024-0147CF46\\IO_SP.lvlib\\K1MP"(w355) -> ()  [unwired: 1 in, 1 out]
    n190 = shared-variable "NI-cRIO9024-0147CF46\\IO_SP.lvlib\\V1MP"(w380) -> ()  [unwired: 1 in, 1 out]
    n191 = shared-variable ".\\IO Library.lvlib\\Pumpe"() -> (w347:bool)  [unwired: 1 in, 1 out]
    n192 = shared-variable "NI-cRIO9024-0147CF46\\IO_SP.lvlib\\PumpOnSP"() -> (w367:bool)  [unwired: 1 in, 1 out]
    n193 = shared-variable "NI-cRIO9024-0147CF46\\IO_SP.lvlib\\PumpOffSP"() -> (w364:bool)  [unwired: 1 in, 1 out]
    n194 = local read "RUCNO/AUTOMATSKI"() -> (w360:bool)
    n195 = local read "Pumpe ON"() -> (w366:bool)
    n196 = local read "Pumpe OFF"() -> (w365:bool)
    n197 = local read "Accept Stop"() -> (w358:bool)
    n198 = shared-variable "NI-cRIO9024-0147CF46\\IO_SP.lvlib\\ASMP"() -> (w359:bool)  [unwired: 1 in, 1 out]
    n199 = shared-variable "NI-cRIO9024-0147CF46\\IO_SP.lvlib\\ARMP"() -> (w361:bool)  [unwired: 1 in, 1 out]
    n200 = shared-variable "NI-cRIO9024-0147CF46\\IO_SP.lvlib\\Pump"(w347) -> ()  [unwired: 1 in, 1 out]
    n201 = Equal?(x=w360, y=w361) -> (x = y?=w363:bool)
    n202 = Equal?(x=w366, y=w367) -> (x = y?=w368:bool)
    n203 = Equal?(x=w358, y=w359) -> (x = y?=w362:bool)
    n204 = Equal?(x=w365, y=w364) -> (x = y?=w369:bool)
    n205 = case shown="False" w363 {
      tunnel: w361 -> [w382 _]
      frame False {
        n206 = property on="RUCNO/AUTOMATSKI" class="Bool (strict)"("Val(Sgnl)"=w382) -> ()  [unwired: 2 in, 2 out]
      }
      frame True {
      }
    }
    n207 = case shown="False" w368 {
      tunnel: w367 -> [w384 _]
      frame False {
        n208 = property on="Pumpe ON" class="Bool (strict)"("Val(Sgnl)"=w384) -> ()  [unwired: 2 in, 2 out]
      }
      frame True {
      }
    }
    n209 = case shown="False" w369 {
      tunnel: w364 -> [w383 _]
      frame False {
        n210 = property on="Pumpe OFF" class="Bool (strict)"("Val(Sgnl)"=w383) -> ()  [unwired: 2 in, 2 out]
      }
      frame True {
      }
    }
    n211 = case shown="False" w362 {
      tunnel: w359 -> [w381 _]
      frame False {
        n212 = property on="Accept Stop" class="Bool (strict)"("Val(Sgnl)"=w381) -> ()  [unwired: 2 in, 2 out]
      }
      frame True {
      }
    }
    n213 = node-c288() -> ()  [unwired: 1 in, 1 out]
  }
  n214 = node-c288(w3) -> ()  [unwired: 1 out]
  n215 = Merge Errors(w8, w7) -> (w6:errorcluster)
  n216 = Release Queue(queue=w9, error in (no error)=w6) -> (error out=w5:errorcluster)  [unwired: 1 in, 2 out]
  n217 = call <vilib>:"Simple Error Handler.vi"("error in (no error)"=w5) -> ()  [unwired: 4 in, 5 out]
